vi "get_config_cluster.vi"(8 "error in (no error)":errorcluster, 11 "GenericPlugin in":refnum<class "LightSourceMG090910LightEmittingDiode.lvclass">) -> (0 "error out":errorcluster, 2 "config cluster (variant)":variant, 3 "GenericPlugin out":refnum<class "LightSourceMG090910LightEmittingDiode.lvclass">)   [LabVIEW 2010, in "LightSourceMG090910LightEmittingDiode.lvclass"]
uses:
  LightSourceMG090910LightEmittingDiode.lvclass
  LightSourceMG090910LightEmittingDiode.lvclass/LightSourceMG090910LightEmittingDiode.ctl
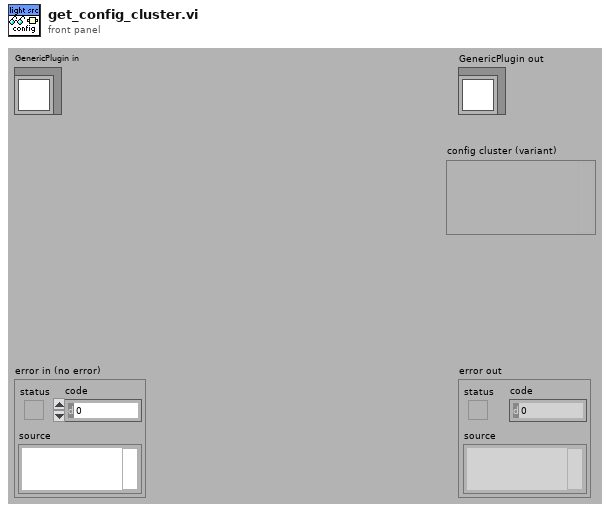
[diagram p1: front panel]
types:
  T1 = typedef "LightSourceMG090910LightEmittingDiode.lvclass/config_data_cluster.ctl" = cluster{"LSID":T2, "manufacturer specification":T3}
  T2 = typedef "LSID_cluster.ctl" = cluster{"identifier":string, "revision":i32}
  T3 = typedef "GenericComponent.lvclass/manufacturer_specification_cluster.ctl" = cluster{"manufacturer":string, "model":string, "serial number":string, "lot number":string}
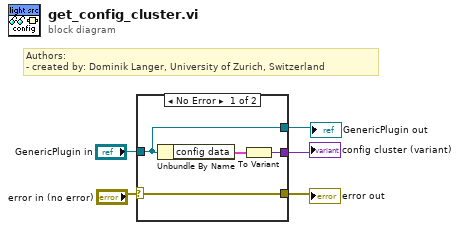
[diagram p0: block diagram]
diagram:
  # "Authors: \n- created by: Dominik Langer, University of Zurich, Switzerland"
  n1 = case shown="No Error" "error in (no error)" {
    selector: "error in (no error)" -> [w6 w10]
    tunnel: "GenericPlugin in" -> [w8 w11]
    tunnel: [w8 w11] -> w1
    tunnel: [w7 _] -> w2
    tunnel: [w6 w10] -> w3
    frame No Error {
      n2 = Unbundle By Name(w8) -> ("config data"=w9:T1)
      n3 = To Variant(anything=w9) -> (Variant=w7:variant)
    }
    frame Error {
    }
  }
  "error out" <- w3
  "GenericPlugin out" <- w1
  "config cluster (variant)" <- w2
